vi "Toggle Active State of Run-Stop Buttons.vi"(4 "inactive button refnum":refnum<vi>, 5 "active button refnum":refnum<vi>, 6 "error in":errorcluster) -> (0 "error out":errorcluster)   [LabVIEW 2020]
doc: "This function will set the active button state to \"Enabled\" and the inactive button state to Disabled and Grayed Out\".\n\nIf the input error status is TRUE (error), then no button attributes are changed."
panel:
  # "Enabled"
  # "Disabled and Grayed Out"
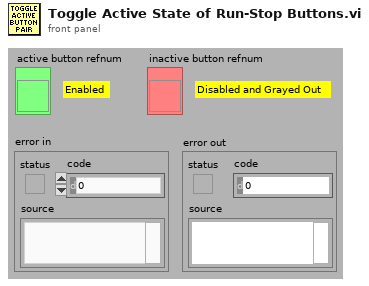
[diagram p1: front panel]
types:
  T1 = enum8{"Enabled", "Disabled", "Disabled and Grayed Out"}
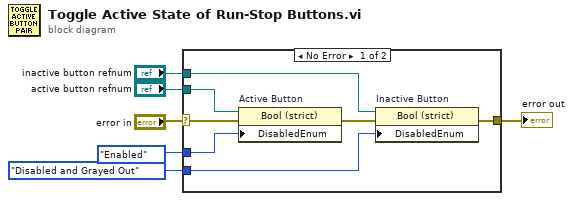
[diagram p0: block diagram]
diagram:
  n1 = case shown="No Error" "error in" {
    selector: "error in" -> [w13 w14]
    tunnel: [w7 w14] -> w6
    tunnel: "active button refnum" -> [w8 _]
    tunnel: "inactive button refnum" -> [w11 _]
    tunnel: T1."Disabled and Grayed Out" ("Disabled") -> [w10 _]
    tunnel: T1."Enabled" ("Disabled") -> [w9 _]
    frame No Error {
      n2 = property on="Active Button" class="Bool (strict)"(reference=w8, error in=w13, "DisabledEnum"=w9) -> (error out=w12:errorcluster)  [unwired: 1 out]
      n3 = property on="Inactive Button" class="Bool (strict)"(reference=w11, error in=w12, "DisabledEnum"=w10) -> (error out=w7:errorcluster)  [unwired: 1 out]
    }
    frame Error {
    }
  }
  "error out" <- w6
